vi "Get Tag.vi"(6 "Namespace":string, 8 "error in (no error)":errorcluster, 10 "Name":string) -> (0 "error out":errorcluster, 1 "found":bool, 2 "Tag Ref out":refnum<data-value>)   [LabVIEW 2018, in "Tag Engine.lvlib" / "Tag Core.lvclass"]
doc: "Lookup the reference of a Tag.\n\nOptionally specify a namespace, which is prepended to the tag name (colon separator).\n\nIf the tag is not found, the found output is false and Error 5602 is returned."
uses:
  Tag Core.lvclass
  Tag/Tag.lvclass
  Tag Core.lvclass/Tag Core.ctl
  <vilib>/Utility/error.llb/Error Cluster From Error Code.vi
  <vilib>/ErrorRing/Error Ring.xnode
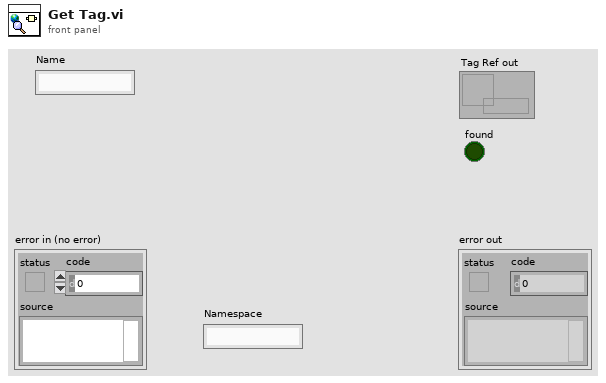
[diagram p1: front panel]
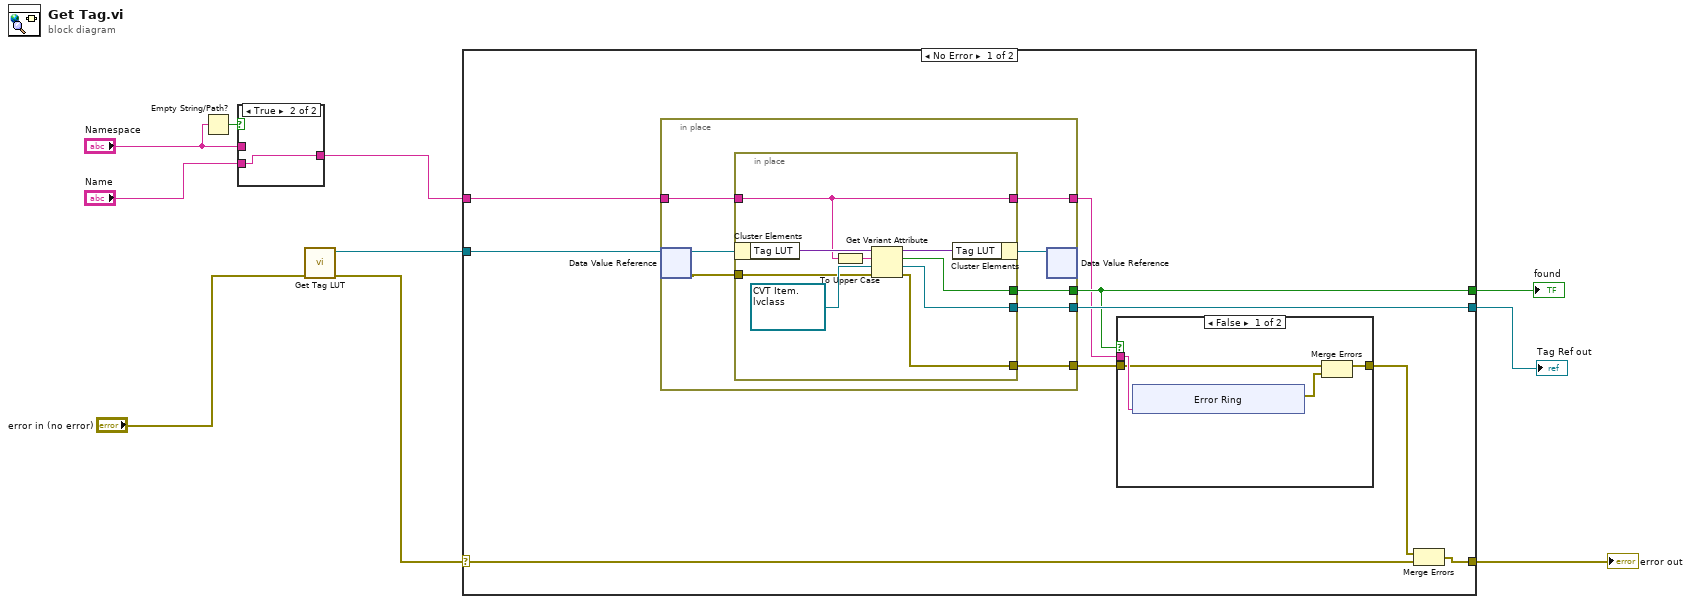
[diagram p0: block diagram]
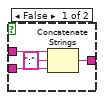
[diagram p2: hidden frame]
diagram:
  n1 = Empty String/Path?(string/path="Namespace") -> (empty?=w7:bool)
  n2 = case shown="True" w7 {
    tunnel: "Namespace" -> [w14 _]
    tunnel: "Name" -> [w12 w15]
    tunnel: [w11 w15] -> w4
    frame False {
      n3 = Concatenate Strings(w14, ":" ("string"), w12) -> (w11:string)
    }
    frame True {
    }
  }
  n4 = call "Get Tag LUT.vi"("error in (no error)"="error in (no error)") -> ("error out"=w2:errorcluster, "Tag LUT Out"=w1:refnum<data-value>)  [unwired: 9 in]
  n5 = case shown="No Error" w2 {
    selector: w2 -> [w19 w54]
    tunnel: [w20 w54] -> w10
    tunnel: w1 -> [w24 _]
    tunnel: [w23 _] -> w8
    tunnel: [w22 _] -> w9
    tunnel: w4 -> [w16 _]
    frame No Error {
      n6 = in-place {
        in-place-border: w16 -> [w43]
        in-place-border: [w42] -> w23
        in-place-border: [w41] -> w22
        in-place-border: [w38] -> w21
        in-place-border: [w37] -> w17
        n7 = in-place-dvr #1(w24) -> (w44:refnum<class "Tag Core.lvclass">, w39:errorcluster)
        n8 = in-place {
          in-place-border: w43 -> [w46]
          in-place-border: [w52] -> w42
          in-place-border: [w50] -> w41
          in-place-border: w39 -> [w48]
          in-place-border: [w47] -> w38
          in-place-border: [w46] -> w37
          n9 = in-place-cluster #2(w44) -> ("Tag LUT"=w53:variant)
          n10 = To Upper Case(1:w46) -> (0:w45:string)
          n11 = Get Variant Attribute(Variant=w53, name=w45, default value (empty Variant)=refnum<data-value> refnum ("CVT Item in"), error in=w48) -> (duplicate Variant=w51:variant, found=w50:bool, value=w52:refnum<data-value>, error out=w47:errorcluster)
          n12 = in-place-cluster #2("Tag LUT"=w51) -> (w40:refnum<class "Tag Core.lvclass">)
        }
        n13 = in-place-dvr #1(w40) -> ()  [unwired: 2 out]
      }
      n14 = case shown="False" w22 {
        tunnel: w21 -> [w27 w36]
        tunnel: [w25 w36] -> w18
        tunnel: w17 -> [w28 _]
        frame False {
          n15 = xnode "Error Ring"("parameter 0"=w28) -> ("error out"=w26:errorcluster)
          n16 = Merge Errors(w27, w26) -> (w25:errorcluster)
        }
        frame True {
        }
      }
      n17 = Merge Errors(w18, w19) -> (w20:errorcluster)
    }
    frame Error {
    }
  }
  "error out" <- w10
  "found" <- w9
  "Tag Ref out" <- w8
